vi "Pick Image.vi"(5 "Image to Add [ ]":T1, 9 "String":string, 11 "error in (no error)":errorcluster) -> (4 "InstanceImage":refnum<k24>, 6 "Valid Image?":bool, 8 "String OUT":string, 10 "Change Font Color?":bool, 15 "error out":errorcluster)   [LabVIEW 2019]
doc: "Version 1.0\nDeveloped by Jean-Marc Simard\nCopyright © 2010, Exaprom Inc.\nAll rights reserved.\nLicense: BSD\n\nWith iTextSharp 4.1.6 (http://itextsharp.sourceforge.net)\nunder Mozilla Public License Version 1.1\n(http://www.mozilla.org/MPL/MPL-1.1.html)"
uses:
  <userlib>/Exaprom PDF/Controls/General Controls/Image to Add refnum [ ].ctl
  C:/Program Files/National Instruments/LabVIEW 2019/user.lib/Exaprom PDF/DLL/itextsharp.dll
  DLL/itextsharp.dll
  <userlib>/Exaprom PDF/VIs/Low level/General/Stop if it True.vi
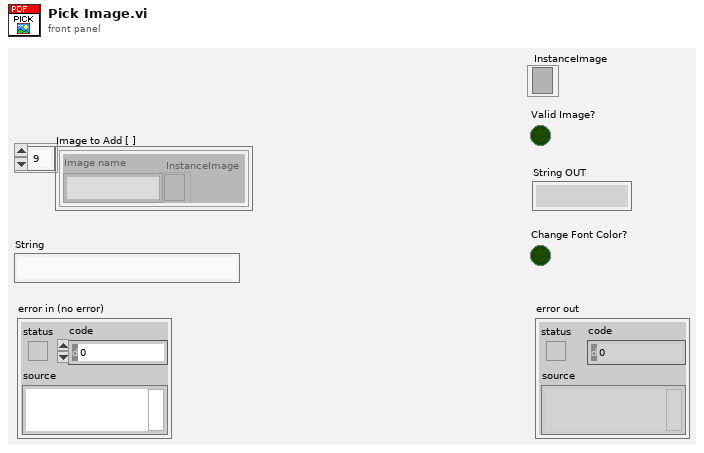
[diagram p1: front panel]
types:
  T1 = typedef "Image to Add refnum [ ].ctl" = cluster{"Image name":string, "InstanceImage":refnum<k24>}[]
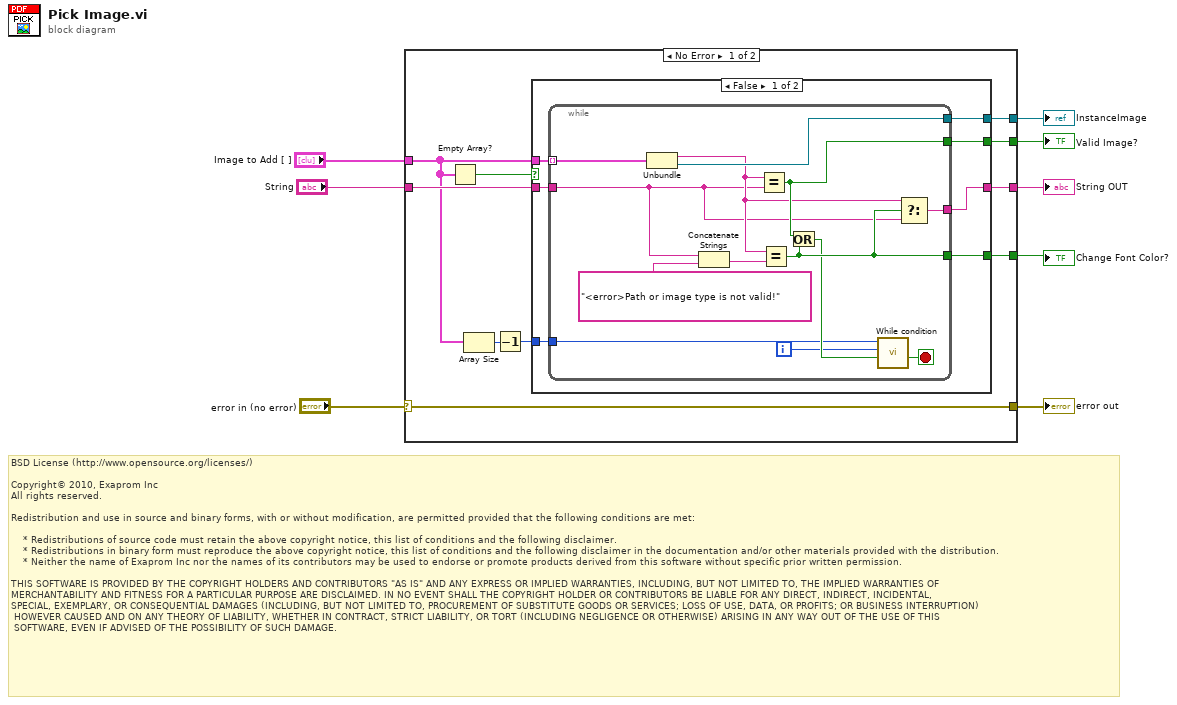
[diagram p0: block diagram]
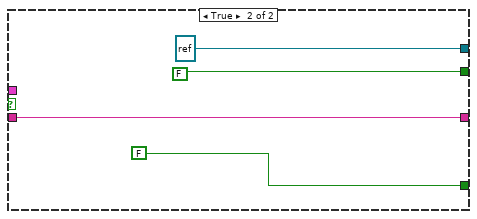
[diagram p2: hidden frame]
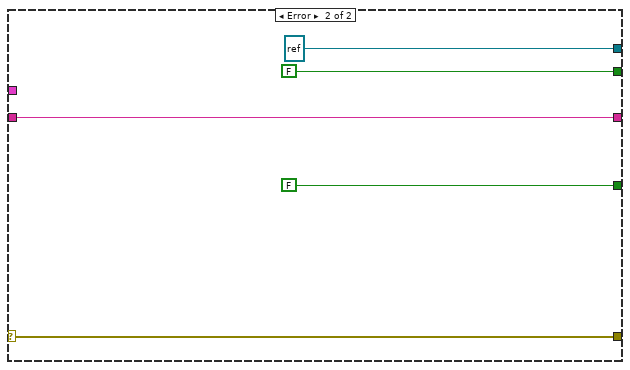
[diagram p3: hidden frame]
diagram:
  # "BSD License (http://www.opensource.org/licenses/)\n\nCopyright© 2010, Exaprom Inc\nAll rights reserved.\n\nRedistribution and use in source and binary forms, with or without modification, are permitted provided that the following conditions are met:\n\n    * Redistributions of source code must retain the above copyright notice, this list of conditions and the following disclaimer.\n    * Redistributions in binary form must reproduce the above copyright notice, this list of conditions and the following disclaimer in the documentation and/or other materials provided with the distribution.\n    * Neither the name of Exaprom Inc nor the names of its contributors may be used to endorse or promote products derived from this software without specific prior written permission.\n\nTHIS SOFTWARE IS PROVIDED BY THE COPYRIGHT HOLDERS AND CONTRIBUTORS \"AS IS\" AND ANY EXPRESS OR IMPLIED WARRANTIES, INCLUDING, BUT NOT LIMITED TO, THE IMPLIED WARRANTIES OF \nMERCHANTABILITY AND FITNESS FOR A PARTICULAR PURPOSE ARE DISCLAIMED. IN NO EVENT SHALL THE COPYRIGHT HOLDER OR CONTRIBUTORS BE LIABLE FOR ANY DIRECT, INDIRECT, INCIDENTAL,\nSPECIAL, EXEMPLARY, OR CONSEQUENTIAL DAMAGES (INCLUDING, BUT NOT LIMITED TO, PROCUREMENT OF SUBSTITUTE GOODS OR SERVICES; LOSS OF USE, DATA, OR PROFITS; OR BUSINESS INTERRUPTION)\n HOWEVER CAUSED AND ON ANY THEORY OF LIABILITY, WHETHER IN CONTRACT, STRICT LIABILITY, OR TORT (INCLUDING NEGLIGENCE OR OTHERWISE) ARISING IN ANY WAY OUT OF THE USE OF THIS\n SOFTWARE, EVEN IF ADVISED OF THE POSSIBILITY OF SUCH DAMAGE."
  n1 = case shown="No Error" "error in (no error)" {
    selector: "error in (no error)" -> [w18 w47]
    tunnel: [w18 w47] -> w8
    tunnel: "Image to Add [ ]" -> [w9 _]
    tunnel: "String" -> [w16 w44]
    tunnel: [w15 refnum<k24> refnum ("InstanceImage")] -> w4
    tunnel: [w12 FALSE] -> w3
    tunnel: [w14 w44] -> w2
    tunnel: [w13 FALSE] -> w1
    frame No Error {
      n2 = Empty Array?(array=w9) -> (empty?=w17:bool)
      n3 = Array Size(array=w9) -> (size(s)=w11:i32)
      n4 = Decrement(x=w11) -> (x-1=w10:i32)
      n5 = case shown="False" w17 {
        tunnel: w16 -> [w21 w39]
        tunnel: w9 -> [w22 _]
        tunnel: [w24 refnum<k24> refnum ("InstanceImage")] -> w15
        tunnel: [w23 FALSE] -> w13
        tunnel: [w20 w39] -> w14
        tunnel: [w25 FALSE] -> w12
        tunnel: w10 -> [w19 _]
        frame False {
          n6 = while {
            tunnel: w22 -> [w38] mode=indexing
            tunnel: w21 -> [w30]
            tunnel: [w37] -> w24
            tunnel: [w32] -> w23
            tunnel: [w34] -> w25
            tunnel: [w33] -> w20
            tunnel: w19 -> [w26]
            i -> [w28]
            stop <- w27 stop-if-true
            n7 = Unbundle(w38) -> ("Image name"=w31:string, "InstanceImage"=w37:refnum<k24>)
            n8 = Concatenate Strings(w30, "<error>Path or image type is not valid!") -> (w35:string)
            n9 = Equal?(x=w31, y=w30) -> (x = y?=w34:bool)
            n10 = Equal?(x=w31, y=w35) -> (x = y?=w32:bool)
            n11 = Or(x=w34, y=w32) -> (x .or. y?=w29:bool)
            n12 = call-poly <userlib>:"While condition.vi"("Test"=w29, "i"=w28, "N"=w26) -> ("Action"=w27:bool)  [unwired: 5 out]
            n13 = Select(t=w31, s=w32, f=w30) -> (s? t:f=w33:string)
          }
        }
        frame True {
        }
      }
    }
    frame Error {
    }
  }
  "error out" <- w8
  "InstanceImage" <- w4
  "Valid Image?" <- w3
  "String OUT" <- w2
  "Change Font Color?" <- w1
